vi "Save.vi"(0 "LV MDI in":refnum<class "LV MDI.lvclass">, 5 "XML File Path":path, 7 "Environment Selection":T1, 11 "error in (no error)":errorcluster) -> (4 "LV MDI out":refnum<class "LV MDI.lvclass">, 15 "error out":errorcluster)   [LabVIEW 2016, in "LV MDI.lvclass"]
uses:
  LV MDI.lvclass
  example/Example1/Typedef/Environment Selection.ctl
  TypeDefs/Data to Save.ctl
  TypeDefs/Set Position.ctl
  LV MDI.lvclass/LV MDI.ctl
  <vilib>/Utility/xml.llb/Write to XML File(string).vi
  Document/Document.lvclass
  Document/Child Classes/LV Doc/LV Doc.lvclass
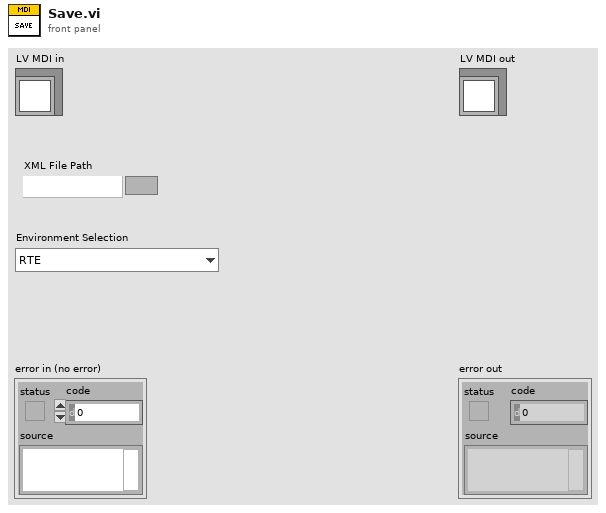
[diagram p1: front panel]
types:
  T1 = typedef "Environment Selection.ctl" = enum16{"RTE", "Dev Environment"}
  T2 = typedef "LV MDI.lvclass/Data to Save.ctl" = cluster{"LV MDI out":refnum<class "LV MDI.lvclass">, "Displayed Doc[]":string[], "Position[]":T3[], "Environment Selection":T1}
  T3 = typedef "LV MDI.lvclass/Set Position.ctl" = cluster{"X":i32, "Y":i32, "Width":i32, "Height":i32}
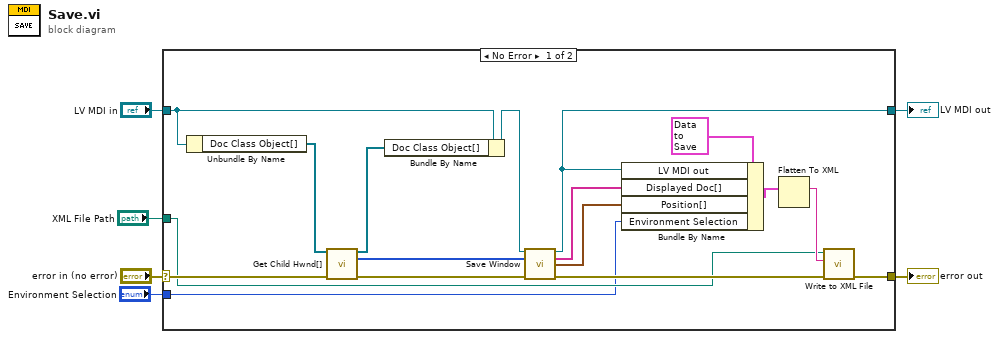
[diagram p0: block diagram]
diagram:
  n1 = case shown="No Error" "error in (no error)" {
    selector: "error in (no error)" -> [w23 w25]
    tunnel: [w11 w25] -> w5
    tunnel: [w15 w24] -> w3
    tunnel: "LV MDI in" -> [w17 w24]
    tunnel: "XML File Path" -> [w8 _]
    tunnel: "Environment Selection" -> [w7 _]
    frame No Error {
      n2 = Unbundle By Name(w17) -> ("Doc Class Object[]"=w22:refnum<class "Document.lvclass">[])
      n3 = call "Get Child Hwnd[].vi"("Doc Class Object[]"=w22, "error in (no error)"=w23) -> ("Doc Class Object[]  2"=w21:refnum<class "Document.lvclass">[], "ChildHwnd[]"=w19:u32[], "error out"=w20:errorcluster)  [unwired: 11 in]
      n4 = Bundle By Name(cluster=w17, "Doc Class Object[]"=w21) -> (w16:refnum<class "LV MDI.lvclass">)
      n5 = call "Save Window.vi"("LV MDI in"=w16, "ChildHwnd[]"=w19, "error in (no error)"=w20) -> ("LV MDI out"=w15:refnum<class "LV MDI.lvclass">, "Displayed Doc[]"=w14:string[], "Position[]"=w13:T3[], "error out"=w9:errorcluster)  [unwired: 9 in]
      n6 = Bundle By Name(cluster=T2 {"LV MDI out"=refnum, "Displayed Doc[]"=["Tank.vi Front Panel"], "Position[]"=[{"X"=586, "Y"=186, "Width"=886, "Height"=486}], "Environment Selection"=enum."RTE"}, "LV MDI out"=w15, "Displayed Doc[]"=w14, "Position[]"=w13, "Environment Selection"=w7) -> (w12:T2)
      n7 = Flatten To XML(anything=w12) -> (xml string=w10:string)
      n8 = call-poly <vilib>:"Write to XML File.vi"("error in (no error)"=w9, "XML Input"=w10, "XML File Path"=w8) -> ("error out"=w11:errorcluster)  [unwired: 6 in, 2 out]
    }
    frame Error {
    }
  }
  "error out" <- w5
  "LV MDI out" <- w3
